vi "Initialize.vi"(4 "Numbers to Exlude":i32[](array[numeric]), 6 "Max Number of Tests":i32, 8 "error in (no error)":errorcluster, 9 "Starting Value":i32, 10 "Name":string, 11 "Test Group in":refnum<class "Test Group.lvclass">) -> (0 "error out":errorcluster, 3 "Test Group out":refnum<class "Test Group.lvclass">)   [LabVIEW 2018, in "Test Number and Bin Generator.lvlib" / "Test Group.lvclass"]
uses:
  Test Group.lvclass
  Test Group.lvclass/Test Group.ctl
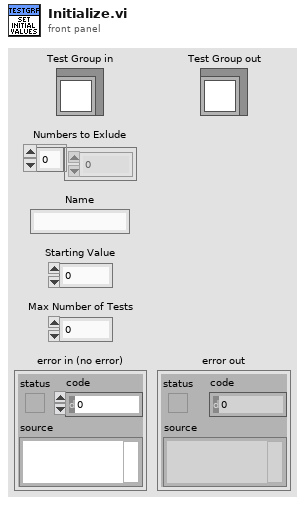
[diagram p1: front panel]
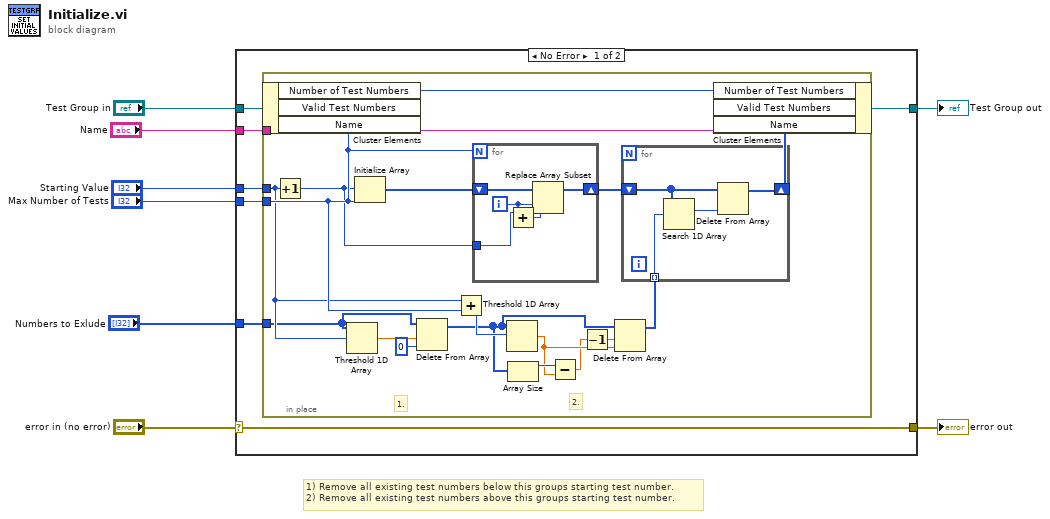
[diagram p0: block diagram]
diagram:
  # "1) Remove all existing test numbers below this groups starting test number.\n2) Remove all existing test numbers above this groups starting test number."
  n1 = case shown="No Error" "error in (no error)" {
    selector: "error in (no error)" -> [w15 w43]
    tunnel: [w15 w43] -> w7
    tunnel: [w10 w42] -> w5
    tunnel: "Test Group in" -> [w11 w42]
    tunnel: "Max Number of Tests" -> [w12 _]
    tunnel: "Starting Value" -> [w13 _]
    tunnel: "Name" -> [w9 _]
    tunnel: "Numbers to Exlude" -> [w14 _]
    frame No Error {
      n2 = in-place {
        in-place-border: w14 -> [w23]
        in-place-border: w13 -> [w24]
        in-place-border: w12 -> [w27]
        in-place-border: w9 -> [w26]
        # "2."
        # "1."
        n3 = in-place-cluster #1(w11) -> ()  [unwired: 3 out]
        n4 = Increment(x=w24) -> (x+1=w25:i32)
        n5 = Threshold 1D Array(2:w24, 3:w23) -> (0:w22:dbl)  [unwired: 1 in]
        n6 = Initialize Array(w25, w27) -> (w32:i32[])
        n7 = Delete From Array(array=w23, length=w22, index=0) -> (array with subset deleted=w20:i32[])  [unwired: 1 out]
        n8 = Add(x=w24, y=w27) -> (x+y=w30:i32)
        n9 = for {
          N: w27 -> [_]
          shift-right: [w40] -> w31
          shift-left: w32 -> [w41]
          tunnel: w25 -> [w37]
          i -> [w39]
          n10 = Add(x=w37, y=w39) -> (x+y=w38:i32)
          n11 = Replace Array Subset(array=w41, new element=w38, index=w39) -> (w40:i32[])
        }
        n12 = Threshold 1D Array(2:w30, 3:w20) -> (0:w18:dbl)  [unwired: 1 in]
        n13 = Array Size(array=w20) -> (size(s)=w19:i32)
        n14 = Subtract(x=w19, y=w18) -> (x-y=w17:dbl)
        n15 = Decrement(x=w17) -> (x-1=w16:dbl)
        n16 = Delete From Array(array=w20, length=w16, index=w18) -> (array with subset deleted=w29:i32[])  [unwired: 1 out]
        n17 = for {
          shift-right: [w34] -> w28
          shift-left: w31 -> [w35]
          tunnel: w29 -> [w36] mode=indexing
          n18 = Search 1D Array(1D array=w35, element=w36) -> (index of element=w33:i32)  [unwired: 1 in]
          n19 = Delete From Array(array=w35, index=w33) -> (array with subset deleted=w34:i32[])  [unwired: 1 in, 1 out]
        }
        n20 = in-place-cluster #1("Number of Test Numbers"=w27, "Valid Test Numbers"=w28, "Name"=w26) -> (w10:refnum<class "Test Group.lvclass">)
      }
    }
    frame Error {
    }
  }
  "error out" <- w7
  "Test Group out" <- w5
